vi "sub_packet_extract.vi"(11 "bitstream":i16[](array[numeric])) -> (0 "Found?":bool, 1 "packet counter":u32, 2 "payload length(bytes)":u32, 3 "payload bytes":u8[](array[numeric]))   [LabVIEW 2014]
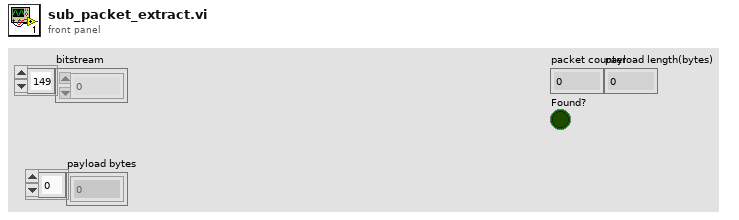
[diagram p1: front panel]
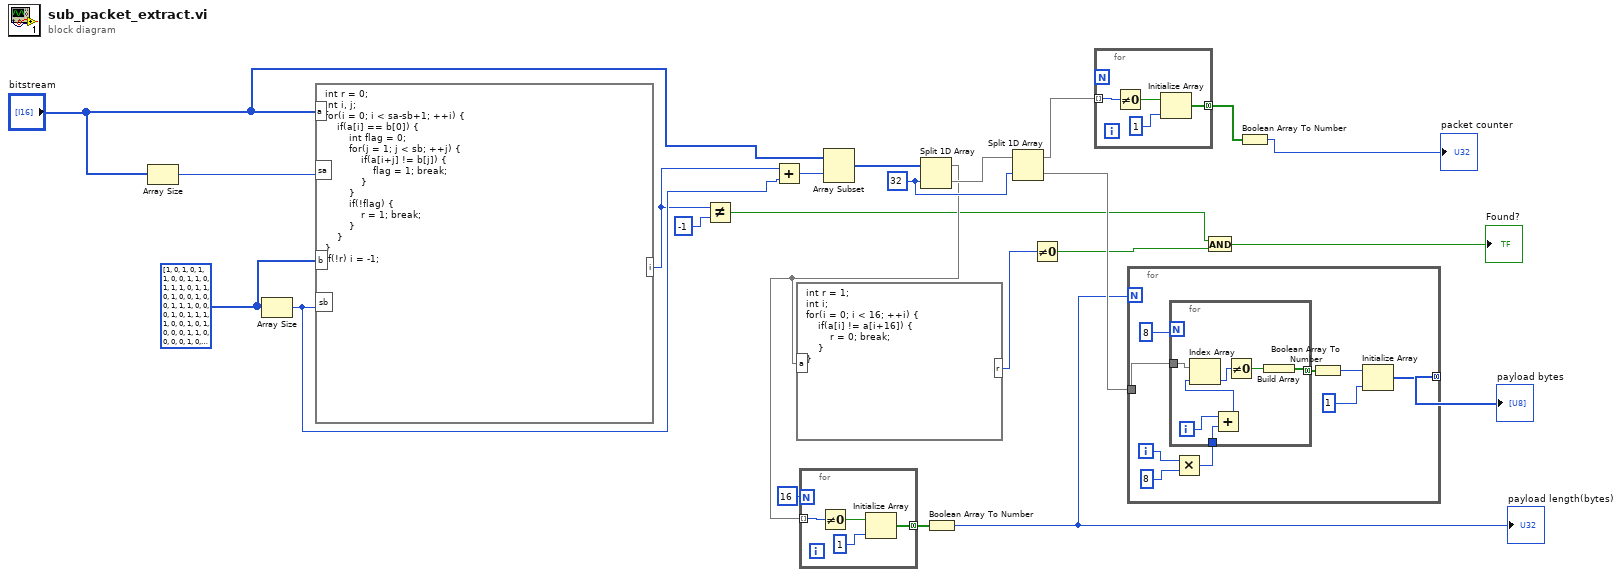
[diagram p0: block diagram]
diagram:
  w1 = i16[] [1, 0, 1, 0, 1, 1, 0, 0, 1, 1, 0, 1, 1, 1, 0, 1, 1, 0, 1, 0, 0, 1, 0, 0, 1, 1, 1, 0, 0, 0, 1, 0, 1, 1, 1, 1, 0, 0, 1, 0, 1, 0, 0, 0, 1, 1, 0, 0, 0, 0, 1, 0, 0, 0, 0, 0, 1, 1, 1, 1, 1, 1, 0, 0] ("preamble(64) 2")
  w16 = 32
  n1 = Array Size(array="bitstream") -> (size(s)=w23:i32)
  n2 = Array Size(array=w1) -> (size(s)=w22:i32)
  n3 = formula code="int r = 0;\nint i, j;\nfor(i = 0; i < sa-sb+1; ++i) {\n    if(a[i] == b[0]) {\n        int flag = 0;\n        for(j = 1; j < sb; ++j) {\n            if(a[i+j] != b[j]) {\n                flag = 1; break;\n            }\n        }\n        if(!flag) {\n            r = 1; break;\n        }\n    }\n}\nif(!r) i = -1;"("b"=w1, "a"="bitstream", "sa"=w23, "sb"=w22) -> ("i"=w21:i32)
  n4 = Not Equal?(x=w21, y=-1) -> (x != y?=w4:bool)
  n5 = Add(x=w21, y=w22) -> (x+y=w7:i32)
  n6 = Array Subset(array="bitstream", index=w7) -> (w19:i16[])  [unwired: 1 in]
  n7 = Split 1D Array(array=w19, index=w16) -> (first subarray=w13:i16[], second subarray=w17:i16[])
  n8 = formula code="int r = 1;\nint i;\nfor(i = 0; i < 16; ++i) {\n    if(a[i] != a[i+16]) {\n        r = 0; break;\n    }\n}"("a"=w13) -> ("r"=w18:i32)
  n9 = for {
    N: 16 -> [_]
    tunnel: w13 -> [w27] mode=indexing
    tunnel: [w25] -> w11 mode=concatenating
    n10 = Not Equal To 0?(x=w27) -> (x != 0?=w26:bool)
    n11 = Initialize Array(w26, 1) -> (w25:bool[])
  }
  n12 = Boolean Array To Number(Boolean array=w11) -> (number=w5:u32)
  "payload length(bytes)" <- w5
  n13 = Split 1D Array(array=w17, index=w16) -> (first subarray=w15:i16[], second subarray=w10:i16[])
  n14 = Not Equal To 0?(x=w18) -> (x != 0?=w3:bool)
  n15 = for {
    tunnel: w15 -> [w31] mode=indexing
    tunnel: [w29] -> w14 mode=concatenating
    n16 = Not Equal To 0?(x=w31) -> (x != 0?=w30:bool)
    n17 = Initialize Array(w30, 1) -> (w29:bool[])
  }
  n18 = for {
    N: w5 -> [_]
    tunnel: w10 -> [w38]
    tunnel: [w36] -> w8 mode=concatenating
    i -> [w34]
    n19 = Multiply(x=w34, y=8) -> (x*y=w32:i32)
    n20 = for {
      N: 8 -> [_]
      tunnel: w38 -> [w42]
      tunnel: [w47] -> w39 mode=concatenating
      tunnel: w32 -> [w44]
      i -> [w45]
      n21 = Add(x=w45, y=w44) -> (x+y=w43:i32)
      n22 = Index Array(array=w42, index=w43) -> (element=w41:i16)
      n23 = Not Equal To 0?(x=w41) -> (x != 0?=w46:bool)
      n24 = Build Array(w46) -> (w47:bool[])
    }
    n25 = Boolean Array To Number(Boolean array=w39) -> (number=w37:u32)
    n26 = Initialize Array(w37, 1) -> (w36:u32[])
  }
  "payload bytes" <- w8
  n27 = And(x=w4, y=w3) -> (x .and. y?=→"Found?":bool)
  n28 = Boolean Array To Number(Boolean array=w14) -> (number=→"packet counter":u32)
